vi "OWC.vi"() -> ()   [LabVIEW 2013]
uses:
  Private/Type Defs/HSB.ctl
  LMH-Hue.lvlib
panel:
  in  "HSB":T1={"Hue"=0, "Saturation"=255, "Brightness"=255}
  in  "Hue":u16
  in  "Stop Button":bool
  in  "Hostname / IP":string="192.168.1.3"
  in  "Username":string="newdeveloper"
  in  "ID":u8=3
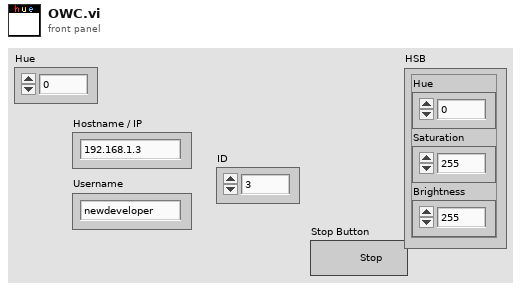
[diagram p1: front panel]
types:
  T1 = typedef "LMH-Hue.lvlib/HSB.ctl" = cluster{"Hue":u16, "Saturation":u8, "Brightness":u8}
  T2 = typedef "LMH-Hue.lvlib/Hue Ref.ctl" = cluster{"HTTP Session":T3, "Base URL":string, "Lights":T4[]}
  T3 = typedef "LabVIEWHTTPClient.lvlib/ClientHandle.ctl" = refnum<k1>
  T4 = typedef "LMH-Hue.lvlib/Light.ctl" = cluster{"ID":i32, "Name":string}
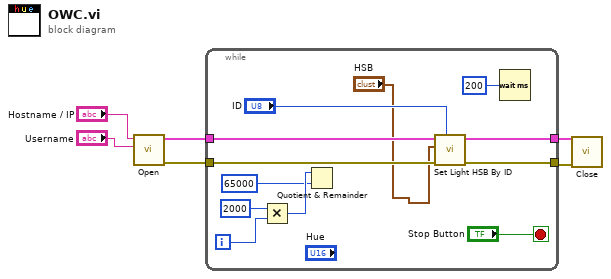
[diagram p0: block diagram]
diagram:
  n1 = call "Open.vi"("Username"="Username", "Hostname / IP"="Hostname / IP") -> ("Error Out"=w5:errorcluster, "Hue Config"=w6:T2)  [unwired: 8 in]
  n2 = while {
    tunnel: w6 -> [w18]
    tunnel: w5 -> [w17]
    tunnel: [w15] -> w1
    tunnel: [w14] -> w2
    i -> [w13]
    stop <- "Stop Button" stop-if-true
    n3 = Multiply(x=2000, y=w13) -> (x*y=w11:i32)
    n4 = Quotient & Remainder(x=w11, y=65000) -> ()  [unwired: 2 out]
    n5 = call "Set Light HSB By ID.vi"("ID"="ID", "Error In"=w17, "HSB"="HSB", "Hue Config"=w18) -> ("Error Out"=w15:errorcluster, "Hue Config"=w14:T2)  [unwired: 6 in]
    n6 = Wait (ms)(milliseconds to wait=u32 200 ("Delay")) -> ()  [unwired: 1 out]
  }
  n7 = call "Close.vi"("Error In"=w1, "Hue Config"=w2) -> ()  [unwired: 9 in, 1 out]
